vi "StopRequest.vi"(8 "error in (no error)":errorcluster, 9 "Wait for Module to stop? (F)":bool, 11 "ModuleAdmin":refnum<class "ModuleAdmin.lvclass">) -> (0 "error out":errorcluster, 2 "Stop Request Sent":bool)   [LabVIEW 2014, in "NetworkImpairmentModule.lvlib"]
uses:
  NetworkImpairmentModule.lvlib
  <userlib>/NIST/ModuleAdminLib/ModuleAdmin/ModuleAdmin.lvclass
  <vilib>/event_ctls.llb/usereventprio.ctl
  PublicAPI/Arguments/Requests/clStopArgument.ctl
  clEventType.ctl
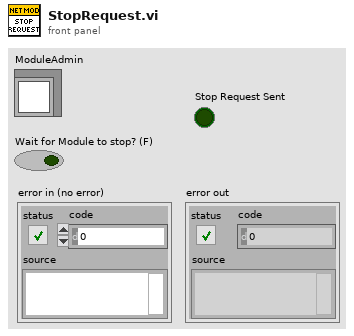
[diagram p1: front panel]
types:
  T1 = typedef "NetworkImpairmentModule.lvlib/clRequestEvents.ctl" = cluster{"StopRequest":refnum<user-event>, "WriteTimeArrayRequest":refnum<user-event>, "WriteNetImpParamsRequest":refnum<user-event>, "ReadNetImpParamsRequest":refnum<user-event>, "WriteLossThresholdRequest":refnum<user-event>, "ReadLossThresholdRequest":refnum<user-event>, "GetNetworkTimeRequest":refnum<user-event>, "GetPktLossRequest":refnum<user-event>, "LoadPluginRequest":refnum<user-event>, "ReadPathToPluginRequest":refnum<user-event>, "ShowPanel":refnum<user-event>}
  T2 = typedef "NetworkImpairmentModule.lvlib/clEventType.ctl" = cluster{"ModuleID":i32, "Data":variant}
  T3 = typedef "NetworkImpairmentModule.lvlib/clStopArgument.ctl" = cluster{"Exit via Stop Module Req?":bool, "Wait for Module to stop?":bool, "ModuleAdmin":refnum<class "ModuleAdmin.lvclass">}
  T4 = typedef "usereventprio.ctl" = enum32{"high priority", "normal priority"}
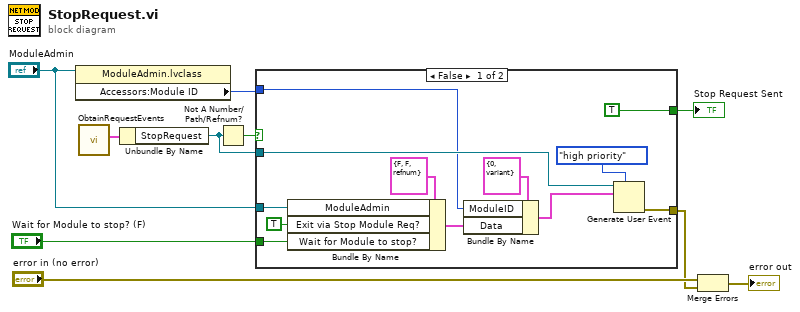
[diagram p0: block diagram]
diagram:
  n1 = property class="ModuleAdmin.lvclass"(reference="ModuleAdmin") -> ("Accessors:Module ID"=w2:i32)  [unwired: 1 in, 2 out]
  n2 = call "ObtainRequestEvents.vi"() -> ("clRequestEvents"=w10:T1)  [unwired: 10 in, 1 out]
  n3 = Unbundle By Name(w10) -> ("StopRequest"=w8:refnum<user-event>)
  n4 = Not A Number/Path/Refnum?(number/path/refnum=w8) -> (NaN/Path/Refnum?=w9:bool)
  n5 = case shown="False" w9 {
    tunnel: w8 -> [w22 _]
    tunnel: w2 -> [w13 _]
    tunnel: "Wait for Module to stop? (F)" -> [w15 _]
    tunnel: [w14 _] -> w4
    tunnel: [TRUE _] -> w3
    tunnel: "ModuleAdmin" -> [w11 _]
    frame False {
      n6 = Bundle By Name(cluster=T3 {"Exit via Stop Module Req?"=FALSE, "Wait for Module to stop?"=FALSE, "ModuleAdmin"=refnum} ("Stop Argument"), "ModuleAdmin"=w11, "Exit via Stop Module Req?"=TRUE, "Wait for Module to stop?"=w15) -> (w17:T3)
      n7 = Bundle By Name(cluster=T2 {"ModuleID"=0, "Data"=variant} ("clBroadcast"), "ModuleID"=w13, "Data"=w17) -> (w16:T2)
      n8 = Generate User Event(priority (normal)=usereventprio."high priority", user event=w22, event data cluster=w16) -> (error out=w14:errorcluster)  [unwired: 1 in, 1 out]
    }
    frame True {
    }
  }
  "Stop Request Sent" <- w3
  n9 = Merge Errors("error in (no error)", w4) -> (→"error out":errorcluster)
